vi "InitShooter.vi"   [LabVIEW 2023]
doc: "This VI initializes miscellaneous devices such as the compressor and any decorations."
uses:
  <vilib>/Rock Robotics/WPI/ThirdParty/Phoenix-LabVIEW/Motor Controller/Controls/CTRE_Phoenix_MotorControl_TalonFXInvertType.ctl
  <vilib>/Rock Robotics/WPI/ThirdParty/Phoenix-LabVIEW/Motor Controller/Controls/CTRE_Phoenix_MotorControl_SupplyCurrentLimitConfiguration.ctl
  <vilib>/Rock Robotics/WPI/ThirdParty/Phoenix-LabVIEW/Motor Controller/Controls/CTRE_Phoenix_MotorControl_LimitSwitchSource_Local.ctl
  <vilib>/Rock Robotics/WPI/ThirdParty/Phoenix-LabVIEW/Motor Controller/Controls/CTRE_Phoenix_MotorControl_LimitSwitchNormal.ctl
  <vilib>/Rock Robotics/WPI/ThirdParty/Phoenix-LabVIEW/Motor Controller/Controls/CTRE_Phoenix_MotorControl_NeutralMode.ctl
  <vilib>/Rock Robotics/WPI/ThirdParty/Phoenix-LabVIEW/Motor Controller/Controls/CTRE_Phoenix_MotorControl_FeedbackDevice_TalonFX.ctl
  <vilib>/Rock Robotics/WPI/ThirdParty/Phoenix-LabVIEW/Motor Controller/Controls/CTRE_Phoenix_MotorControl_StatusFrameEnhanced.ctl
  GlobalShooter.vi
  <vilib>/Rock Robotics/WPI/Solenoid/WPI_SolenoidChannel.ctl
  <vilib>/Rock Robotics/WPI/Solenoid/WPI_SolenoidOpenDouble.vi
types:
  T1 = typedef "CTRE_Phoenix_MotorControl_StatusFrameEnhanced.ctl" = u16
  T2 = typedef "CTRE_Phoenix_MotorControl_SupplyCurrentLimitConfiguration.ctl" = cluster{"Enable?":bool, "Current Limit":dbl, "Threshold Current":dbl, "Threshold Time":dbl}
  T3 = typedef "CTRE_Phoenix_MotorControl_FeedbackDevice_TalonFX.ctl" = i8
  T4 = typedef "CTRE_Phoenix_MotorControl_NeutralMode.ctl" = enum8{"EEPROMSetting", "Override to Coast", "Override to Brake"}
  T5 = typedef "CTRE_Phoenix_MotorControl_TalonFXInvertType.ctl" = enum16{"Counter-Clockwise", "Clockwise"}
  T6 = typedef "CTRE_Phoenix_MotorControl_LimitSwitchNormal.ctl" = enum16{"Normally Open", "Normally Closed", "Disabled"}
  T7 = typedef "CTRE_Phoenix_MotorControl_LimitSwitchSource_Local.ctl" = enum16{"Feedback Connector", "Remote Talon SRX", "Remote CANifier", "Deactivated"}
  T8 = typedef "WPI_SolenoidChannel.ctl" = enum8{"Solenoid 0", "Solenoid 1", "Solenoid 2", "Solenoid 3", "Solenoid 4", "Solenoid 5", "Solenoid 6", "Solenoid 7", "Solenoid 8", "Solenoid 9", "Solenoid 10", "Solenoid 11", "Solenoid 12", "Solenoid 13", "Solenoid 14", "Solenoid 15", "Invalid"}
  T9 = typedef "WPI_SolenoidDevRef.ctl" = cluster{"DevStatus":errorcluster, "Pneumatics Control Module":u8, "Forward Solenoid Channel":T8, "Reverse Solenoid Channel":T8}
  T10 = typedef "WPI_MotorControlDeviceRef.ctl" = cluster{"DeviceStatus":errorcluster, "Type":T11, "PWM":cluster{"PWM Channel":T12, "DeadBand":T13}, "CAN":cluster{"Device Number":u8, "SetOutput VI Ref":variant, "GetOutput VI Ref":variant, "Enable VI Ref":variant, "Disable VI Ref":variant, "Data":variant}, "Invert":bool, "DIO PWM":cluster{"PWM \"Enable\" Channel":T12, "DIOChannel":T14, "PWM Rate":dbl}}
  T11 = typedef "WPI_MotorControlType.ctl" = enum16{"PWM", "CAN", "DIO PWM"}
  T12 = typedef "FPGA_DIOPWMChannel.ctl" = enum8{"PWM 0", "PWM 1", "PWM 2", "PWM 3", "PWM 4", "PWM 5", "PWM 6", "PWM 7", "PWM 8", "PWM 9", "PWM MXP 0", "PWM MXP 1", "PWM MXP 2", "PWM MXP 3", "PWM MXP 4", "PWM MXP 5", "PWM MXP 6", "PWM MXP 7", "PWM MXP 8", "PWM MXP 9", "Invalid"}
  T13 = typedef "WPI_PWMDeadband.ctl" = cluster{"Name":string, "maxPositivePwm":i32, "minPositivePwm":i32, "centerPwm":i32, "maxNegativePwm":i32, "minNegativePwm":i32, "angularRange":u16}
  T14 = typedef "FPGA_DIOChannel.ctl" = enum8{"DIO 0", "DIO 1", "DIO 2", "DIO 3", "DIO 4", "DIO 5", "DIO 6", "DIO 7", "DIO 8", "DIO 9", "DIO MXP 0", "DIO MXP 1", "DIO MXP 2", "DIO MXP 3", "DIO MXP 4", "DIO MXP 5", "DIO MXP 6", "DIO MXP 7", "DIO MXP 8", "DIO MXP 9", "DIO MXP 10", "DIO MXP 11", "DIO MXP 12", "DIO MXP 13", "DIO MXP 14", "DIO MXP 15", "SPI Port CS1", "SPI Port CS2", "SPI Port CS3", "SPI Port MISO", "SPI Port MOSI", "Invalid"}
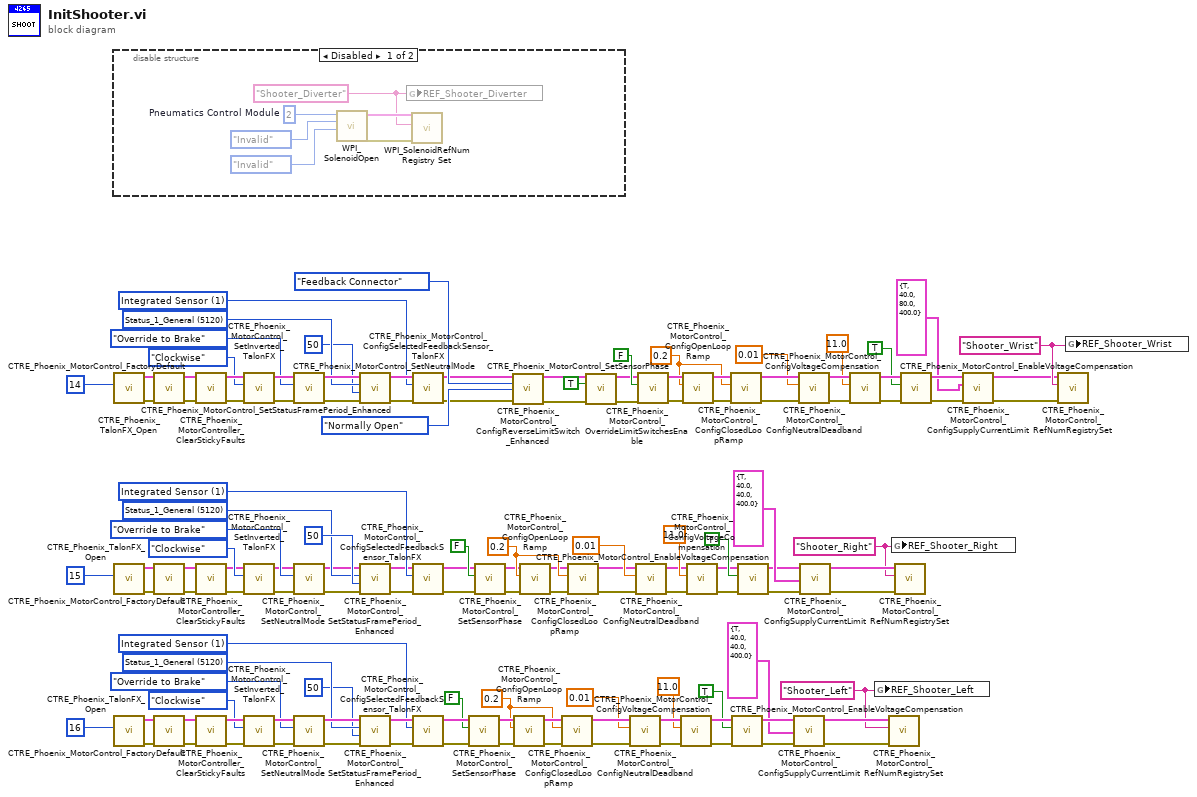
[diagram p0: block diagram]
diagram:
  w7 = "Shooter_Left" ("refnum name")
  w18 = T1 5120 items=["Status_1_General"=5120, "Status_2_Feedback0"=5184, "Status_3_Quadrature"=5248, "Status_4_AinTempVbat"=5312, "Status_6_Misc"=5440, "Status_7_CommStatus"=5504, "Status_8_PulseWidth"=5568, "Status_9_MotProfBuffer"=5632, "Status_10_MotionMagic"=5696, "Status_11_UartGadgeteer"=5760, "Status_12_Feedback1"=5824, "Status_13_Base_PIDF0"=5888, "Status_14_Turn_PIDF1"=5952, "Status_15_FirmwareApiStatus"=6016, "Status_Brushless_Current"=4672] ("Status Frame")
  w14 = 0.2 ("secondsFromNeutralToFull")
  w16 = T3 1 items=["Integrated Sensor"=1, "Sensor Sum (S0 + S1)"=9, "Sensor Difference (D0 - D1)"=10, "Remote Source 0"=11, "Remote Source 1"=12, "None"=14, "Software Emulated"=15] ("Talon FX Feedback Device")
  w50 = "Shooter_Right" ("refnum name")
  w78 = T1 5120 items=["Status_1_General"=5120, "Status_2_Feedback0"=5184, "Status_3_Quadrature"=5248, "Status_4_AinTempVbat"=5312, "Status_6_Misc"=5440, "Status_7_CommStatus"=5504, "Status_8_PulseWidth"=5568, "Status_9_MotProfBuffer"=5632, "Status_10_MotionMagic"=5696, "Status_11_UartGadgeteer"=5760, "Status_12_Feedback1"=5824, "Status_13_Base_PIDF0"=5888, "Status_14_Turn_PIDF1"=5952, "Status_15_FirmwareApiStatus"=6016, "Status_Brushless_Current"=4672] ("Status Frame")
  w82 = 0.2 ("secondsFromNeutralToFull")
  w80 = T3 1 items=["Integrated Sensor"=1, "Sensor Sum (S0 + S1)"=9, "Sensor Difference (D0 - D1)"=10, "Remote Source 0"=11, "Remote Source 1"=12, "None"=14, "Software Emulated"=15] ("Talon FX Feedback Device")
  w103 = T1 5120 items=["Status_1_General"=5120, "Status_2_Feedback0"=5184, "Status_3_Quadrature"=5248, "Status_4_AinTempVbat"=5312, "Status_6_Misc"=5440, "Status_7_CommStatus"=5504, "Status_8_PulseWidth"=5568, "Status_9_MotProfBuffer"=5632, "Status_10_MotionMagic"=5696, "Status_11_UartGadgeteer"=5760, "Status_12_Feedback1"=5824, "Status_13_Base_PIDF0"=5888, "Status_14_Turn_PIDF1"=5952, "Status_15_FirmwareApiStatus"=6016, "Status_Brushless_Current"=4672] ("Status Frame")
  w94 = "Shooter_Wrist" ("refnum name")
  w99 = 0.2 ("secondsFromNeutralToFull")
  w101 = T3 1 items=["Integrated Sensor"=1, "Sensor Sum (S0 + S1)"=9, "Sensor Difference (D0 - D1)"=10, "Remote Source 0"=11, "Remote Source 1"=12, "None"=14, "Software Emulated"=15] ("Talon FX Feedback Device")
  n1 = disable-structure shown="Disabled" {
    frame Disabled {
      w131 = "Shooter_Diverter" ("refnum name")
      w136 = u8 2  # Pneumatics Control Module
      n2 = call-poly <vilib>:"WPI_SolenoidOpen.vi"("Reverse Solenoid Channel"=WPI_SolenoidChannel."Invalid", "Forward Solenoid Channel"=WPI_SolenoidChannel."Invalid", "Pneumatics Device (def)"=w136) -> ("error out"=w132:errorcluster, "SolenoidDevRef"=w133:T9)  [unwired: 7 in]
      n3 = global write "GlobalShooter.vi" "REF_Shooter_Diverter"(w131) -> ()
      n4 = call <vilib>:"WPI_SolenoidRefNum Registry Set.vi"("error in (no error)"=w132, "refnum name"=w131, "SolenoidDevRef"=w133) -> ()  [unwired: 7 in, 2 out]
    }
    frame Enabled {
    }
  }
  n5 = call <vilib>:"CTRE_Phoenix_TalonFX_Open.vi"("Device Number"=u8 14) -> ("error out"=w115:errorcluster, "PhoenixMotorControlDevRef"=w123:T10)  [unwired: 9 in]
  n6 = call <vilib>:"CTRE_Phoenix_TalonFX_Open.vi"("Device Number"=u8 15) -> ("error out"=w66:errorcluster, "PhoenixMotorControlDevRef"=w58:T10)  [unwired: 9 in]
  n7 = call <vilib>:"CTRE_Phoenix_TalonFX_Open.vi"("Device Number"=u8 16) -> ("error out"=w30:errorcluster, "PhoenixMotorControlDevRef"=w38:T10)  [unwired: 9 in]
  n8 = call <vilib>:"CTRE_Phoenix_MotorControl_FactoryDefault.vi"("error in"=w115, "PhoenixMotorControlDevRef"=w123) -> ("error out"=w116:errorcluster, "PhoenixMotorControlDevRef"=w124:T10)  [unwired: 8 in]
  n9 = call <vilib>:"CTRE_Phoenix_MotorControl_FactoryDefault.vi"("error in"=w66, "PhoenixMotorControlDevRef"=w58) -> ("error out"=w65:errorcluster, "PhoenixMotorControlDevRef"=w57:T10)  [unwired: 8 in]
  n10 = call <vilib>:"CTRE_Phoenix_MotorControl_FactoryDefault.vi"("error in"=w30, "PhoenixMotorControlDevRef"=w38) -> ("error out"=w31:errorcluster, "PhoenixMotorControlDevRef"=w39:T10)  [unwired: 8 in]
  n11 = call <vilib>:"CTRE_Phoenix_MotorController_ClearStickyFaults.vi"("error in"=w116, "PhoenixMotorControlDevRef"=w124) -> ("error out"=w117:errorcluster, "PhoenixMotorControlDevRef"=w125:T10)  [unwired: 8 in]
  n12 = call <vilib>:"CTRE_Phoenix_MotorController_ClearStickyFaults.vi"("error in"=w65, "PhoenixMotorControlDevRef"=w57) -> ("error out"=w64:errorcluster, "PhoenixMotorControlDevRef"=w56:T10)  [unwired: 8 in]
  n13 = call <vilib>:"CTRE_Phoenix_MotorController_ClearStickyFaults.vi"("error in"=w31, "PhoenixMotorControlDevRef"=w39) -> ("error out"=w32:errorcluster, "PhoenixMotorControlDevRef"=w40:T10)  [unwired: 8 in]
  n14 = call <vilib>:"CTRE_Phoenix_MotorControl_SetInverted_TalonFX.vi"("error in (no error)"=w117, "Invert Type"=CTRE_Phoenix_MotorControl_TalonFXInvertType."Clockwise", "PhoenixMotorControlDevRef"=w125) -> ("error out"=w118:errorcluster, "PhoenixMotorControlDevRef"=w126:T10)  [unwired: 7 in]
  n15 = call <vilib>:"CTRE_Phoenix_MotorControl_SetInverted_TalonFX.vi"("error in (no error)"=w64, "Invert Type"=CTRE_Phoenix_MotorControl_TalonFXInvertType."Clockwise", "PhoenixMotorControlDevRef"=w56) -> ("error out"=w63:errorcluster, "PhoenixMotorControlDevRef"=w55:T10)  [unwired: 7 in]
  n16 = call <vilib>:"CTRE_Phoenix_MotorControl_SetInverted_TalonFX.vi"("error in (no error)"=w32, "Invert Type"=CTRE_Phoenix_MotorControl_TalonFXInvertType."Clockwise", "PhoenixMotorControlDevRef"=w40) -> ("error out"=w33:errorcluster, "PhoenixMotorControlDevRef"=w41:T10)  [unwired: 7 in]
  n17 = call <vilib>:"CTRE_Phoenix_MotorControl_SetNeutralMode.vi"("error in (no error)"=w118, "Motor Control Neutral Mode"=CTRE_Phoenix_MotorControl_NeutralMode."Override to Brake", "PhoenixMotorControlDevRef"=w126) -> ("error out"=w119:errorcluster, "PhoenixMotorControlDevRef"=w130:T10)  [unwired: 7 in]
  n18 = call <vilib>:"CTRE_Phoenix_MotorControl_SetNeutralMode.vi"("error in (no error)"=w63, "Motor Control Neutral Mode"=CTRE_Phoenix_MotorControl_NeutralMode."Override to Brake", "PhoenixMotorControlDevRef"=w55) -> ("error out"=w62:errorcluster, "PhoenixMotorControlDevRef"=w51:T10)  [unwired: 7 in]
  n19 = call <vilib>:"CTRE_Phoenix_MotorControl_SetNeutralMode.vi"("error in (no error)"=w33, "Motor Control Neutral Mode"=CTRE_Phoenix_MotorControl_NeutralMode."Override to Brake", "PhoenixMotorControlDevRef"=w41) -> ("error out"=w34:errorcluster, "PhoenixMotorControlDevRef"=w45:T10)  [unwired: 7 in]
  n20 = call <vilib>:"CTRE_Phoenix_MotorControl_SetStatusFramePeriod_Enhanced.vi"("error in (no error)"=w119, "periodMs"=50, "Status Frame"=w103, "PhoenixMotorControlDevRef"=w130) -> ("error out"=w120:errorcluster, "PhoenixMotorControlDevRef"=w121:T10)  [unwired: 6 in]
  n21 = call <vilib>:"CTRE_Phoenix_MotorControl_SetStatusFramePeriod_Enhanced.vi"("error in (no error)"=w62, "periodMs"=50, "Status Frame"=w78, "PhoenixMotorControlDevRef"=w51) -> ("error out"=w61:errorcluster, "PhoenixMotorControlDevRef"=w60:T10)  [unwired: 6 in]
  n22 = call <vilib>:"CTRE_Phoenix_MotorControl_SetStatusFramePeriod_Enhanced.vi"("error in (no error)"=w34, "periodMs"=50, "Status Frame"=w18, "PhoenixMotorControlDevRef"=w45) -> ("error out"=w35:errorcluster, "PhoenixMotorControlDevRef"=w36:T10)  [unwired: 6 in]
  n23 = call <vilib>:"CTRE_Phoenix_MotorControl_ConfigSelectedFeedbackSensor_TalonFX.vi"("error in (no error)"=w120, "Talon FX Feedback Device"=w101, "PhoenixMotorControlDevRef"=w121) -> ("error out"=w1:errorcluster, "PhoenixMotorControlDevRef"=w2:T10)  [unwired: 7 in]
  n24 = call <vilib>:"CTRE_Phoenix_MotorControl_ConfigSelectedFeedbackSensor_TalonFX.vi"("error in (no error)"=w61, "Talon FX Feedback Device"=w80, "PhoenixMotorControlDevRef"=w60) -> ("error out"=w48:errorcluster, "PhoenixMotorControlDevRef"=w49:T10)  [unwired: 7 in]
  n25 = call <vilib>:"CTRE_Phoenix_MotorControl_ConfigSelectedFeedbackSensor_TalonFX.vi"("error in (no error)"=w35, "Talon FX Feedback Device"=w16, "PhoenixMotorControlDevRef"=w36) -> ("error out"=w47:errorcluster, "PhoenixMotorControlDevRef"=w46:T10)  [unwired: 7 in]
  n26 = call <vilib>:"CTRE_Phoenix_MotorControl_SetSensorPhase.vi"("error in (no error)"=w47, "PhaseSensor"=FALSE, "PhoenixMotorControlDevRef"=w46) -> ("error out"=w25:errorcluster, "PhoenixMotorControlDevRef"=w26:T10)  [unwired: 7 in]
  n27 = call <vilib>:"CTRE_Phoenix_MotorControl_SetSensorPhase.vi"("error in (no error)"=w48, "PhaseSensor"=FALSE, "PhoenixMotorControlDevRef"=w49) -> ("error out"=w71:errorcluster, "PhoenixMotorControlDevRef"=w70:T10)  [unwired: 7 in]
  n28 = call <vilib>:"CTRE_Phoenix_MotorControl_ConfigReverseLimitSwitch_Enhanced.vi"("PhoenixMotorControlDevRef"=w2, "Limit Switch Source"=CTRE_Phoenix_MotorControl_LimitSwitchSource_Local."Feedback Connector", "NormallyOpenOrClosed"=CTRE_Phoenix_MotorControl_LimitSwitchNormal."Normally Open", "error in (no error)"=w1) -> ("PhoenixMotorControlDevRef"=w4:T10, "error out"=w3:errorcluster)  [unwired: 10 in]
  n29 = call <vilib>:"CTRE_Phoenix_MotorControl_ConfigOpenLoopRamp.vi"("error in (no error)"=w25, "secondsFromNeutralToFull"=w14, "PhoenixMotorControlDevRef"=w26) -> ("error out"=w29:errorcluster, "PhoenixMotorControlDevRef"=w42:T10)  [unwired: 7 in]
  n30 = call <vilib>:"CTRE_Phoenix_MotorControl_ConfigOpenLoopRamp.vi"("error in (no error)"=w71, "secondsFromNeutralToFull"=w82, "PhoenixMotorControlDevRef"=w70) -> ("error out"=w67:errorcluster, "PhoenixMotorControlDevRef"=w54:T10)  [unwired: 7 in]
  n31 = call <vilib>:"CTRE_Phoenix_MotorControl_ConfigClosedLoopRamp.vi"("error in (no error)"=w29, "secondsFromNeutralToFull"=w14, "PhoenixMotorControlDevRef"=w42) -> ("error out"=w23:errorcluster, "PhoenixMotorControlDevRef"=w24:T10)  [unwired: 7 in]
  n32 = call <vilib>:"CTRE_Phoenix_MotorControl_ConfigClosedLoopRamp.vi"("error in (no error)"=w67, "secondsFromNeutralToFull"=w82, "PhoenixMotorControlDevRef"=w54) -> ("error out"=w73:errorcluster, "PhoenixMotorControlDevRef"=w72:T10)  [unwired: 7 in]
  n33 = call <vilib>:"CTRE_Phoenix_MotorControl_OverrideLimitSwitchesEnable.vi"("PhoenixMotorControlDevRef"=w4, "Override Limit Switch Enable?"=TRUE, "error in (no error)"=w3) -> ("PhoenixMotorControlDevRef"=w91:T10, "error out"=w90:errorcluster)  [unwired: 11 in]
  n34 = call <vilib>:"CTRE_Phoenix_MotorControl_ConfigNeutralDeadband.vi"("error in (no error)"=w23, "Percent Deadband"=0.01, "PhoenixMotorControlDevRef"=w24) -> ("error out"=w22:errorcluster, "PhoenixMotorControlDevRef"=w21:T10)  [unwired: 7 in]
  n35 = call <vilib>:"CTRE_Phoenix_MotorControl_ConfigNeutralDeadband.vi"("error in (no error)"=w73, "Percent Deadband"=0.01, "PhoenixMotorControlDevRef"=w72) -> ("error out"=w74:errorcluster, "PhoenixMotorControlDevRef"=w75:T10)  [unwired: 7 in]
  n36 = call <vilib>:"CTRE_Phoenix_MotorControl_SetSensorPhase.vi"("error in (no error)"=w90, "PhaseSensor"=FALSE, "PhoenixMotorControlDevRef"=w91) -> ("error out"=w110:errorcluster, "PhoenixMotorControlDevRef"=w111:T10)  [unwired: 7 in]
  n37 = call <vilib>:"CTRE_Phoenix_MotorControl_ConfigVoltageCompensation.vi"("error in (no error)"=w22, "Saturation Voltage"=11.0, "PhoenixMotorControlDevRef"=w21) -> ("error out"=w28:errorcluster, "PhoenixMotorControlDevRef"=w43:T10)  [unwired: 7 in]
  n38 = call <vilib>:"CTRE_Phoenix_MotorControl_ConfigOpenLoopRamp.vi"("error in (no error)"=w110, "secondsFromNeutralToFull"=w99, "PhoenixMotorControlDevRef"=w111) -> ("error out"=w114:errorcluster, "PhoenixMotorControlDevRef"=w127:T10)  [unwired: 7 in]
  n39 = call <vilib>:"CTRE_Phoenix_MotorControl_ConfigVoltageCompensation.vi"("error in (no error)"=w74, "Saturation Voltage"=11.0, "PhoenixMotorControlDevRef"=w75) -> ("error out"=w68:errorcluster, "PhoenixMotorControlDevRef"=w53:T10)  [unwired: 7 in]
  n40 = call <vilib>:"CTRE_Phoenix_MotorControl_ConfigClosedLoopRamp.vi"("error in (no error)"=w114, "secondsFromNeutralToFull"=w99, "PhoenixMotorControlDevRef"=w127) -> ("error out"=w108:errorcluster, "PhoenixMotorControlDevRef"=w109:T10)  [unwired: 7 in]
  n41 = call <vilib>:"CTRE_Phoenix_MotorControl_EnableVoltageCompensation.vi"("error in (no error)"=w28, "Enable Voltage Compensation?"=TRUE, "PhoenixMotorControlDevRef"=w43) -> ("error out"=w27:errorcluster, "PhoenixMotorControlDevRef"=w44:T10)  [unwired: 7 in]
  n42 = call <vilib>:"CTRE_Phoenix_MotorControl_EnableVoltageCompensation.vi"("error in (no error)"=w68, "Enable Voltage Compensation?"=TRUE, "PhoenixMotorControlDevRef"=w53) -> ("error out"=w69:errorcluster, "PhoenixMotorControlDevRef"=w52:T10)  [unwired: 7 in]
  n43 = call <vilib>:"CTRE_Phoenix_MotorControl_ConfigSupplyCurrentLimit.vi"("error in (no error)"=w27, "Supply Current Limit Configuration"=T2 {"Enable?"=TRUE, "Current Limit"=40.0, "Threshold Current"=40.0, "Threshold Time"=400.0}, "PhoenixMotorControlDevRef"=w44) -> ("error out"=w8:errorcluster, "PhoenixMotorControlDevRef"=w9:T10)  [unwired: 7 in]
  n44 = call <vilib>:"CTRE_Phoenix_MotorControl_ConfigNeutralDeadband.vi"("error in (no error)"=w108, "Percent Deadband"=0.01, "PhoenixMotorControlDevRef"=w109) -> ("error out"=w107:errorcluster, "PhoenixMotorControlDevRef"=w106:T10)  [unwired: 7 in]
  n45 = call <vilib>:"CTRE_Phoenix_MotorControl_ConfigSupplyCurrentLimit.vi"("error in (no error)"=w69, "Supply Current Limit Configuration"=T2 {"Enable?"=TRUE, "Current Limit"=40.0, "Threshold Current"=40.0, "Threshold Time"=400.0}, "PhoenixMotorControlDevRef"=w52) -> ("error out"=w88:errorcluster, "PhoenixMotorControlDevRef"=w87:T10)  [unwired: 7 in]
  n46 = call <vilib>:"CTRE_Phoenix_MotorControl_ConfigVoltageCompensation.vi"("error in (no error)"=w107, "Saturation Voltage"=11.0, "PhoenixMotorControlDevRef"=w106) -> ("error out"=w113:errorcluster, "PhoenixMotorControlDevRef"=w128:T10)  [unwired: 7 in]
  n47 = global write "GlobalShooter.vi" "REF_Shooter_Left"(w7) -> ()
  n48 = call <vilib>:"CTRE_Phoenix_MotorControl_RefNumRegistrySet.vi"("error in (no error)"=w8, "refnum name"=w7, "PhoenixMotorControlDevRef"=w9) -> ()  [unwired: 7 in, 2 out]
  n49 = global write "GlobalShooter.vi" "REF_Shooter_Right"(w50) -> ()
  n50 = call <vilib>:"CTRE_Phoenix_MotorControl_RefNumRegistrySet.vi"("error in (no error)"=w88, "refnum name"=w50, "PhoenixMotorControlDevRef"=w87) -> ()  [unwired: 7 in, 2 out]
  n51 = call <vilib>:"CTRE_Phoenix_MotorControl_EnableVoltageCompensation.vi"("error in (no error)"=w113, "Enable Voltage Compensation?"=TRUE, "PhoenixMotorControlDevRef"=w128) -> ("error out"=w112:errorcluster, "PhoenixMotorControlDevRef"=w129:T10)  [unwired: 7 in]
  n52 = call <vilib>:"CTRE_Phoenix_MotorControl_ConfigSupplyCurrentLimit.vi"("error in (no error)"=w112, "Supply Current Limit Configuration"=T2 {"Enable?"=TRUE, "Current Limit"=40.0, "Threshold Current"=80.0, "Threshold Time"=400.0}, "PhoenixMotorControlDevRef"=w129) -> ("error out"=w92:errorcluster, "PhoenixMotorControlDevRef"=w93:T10)  [unwired: 7 in]
  n53 = call <vilib>:"CTRE_Phoenix_MotorControl_RefNumRegistrySet.vi"("error in (no error)"=w92, "refnum name"=w94, "PhoenixMotorControlDevRef"=w93) -> ()  [unwired: 7 in, 2 out]
  n54 = global write "GlobalShooter.vi" "REF_Shooter_Wrist"(w94) -> ()
